vi "Dashboard Main.vi"() -> ()   [LabVIEW 2015]
uses:
  <vilib>/Utility/miscctls.llb/LVRowAndColumnTypeDef.ctl
  <vilib>/event_ctls.llb/eventvkey.ctl
  <vilib>/Rock Robotics/WPI/Dashboard/WPI_DashboardLogging Global.vi
  <vilib>/Rock Robotics/Network Tables/NT Read Numeric Array.vi
  <vilib>/Utility/config.llb/Write Key (String).vi
  <vilib>/Utility/config.llb/Write Key (I32).vi
  <vilib>/Utility/config.llb/NI_LVConfig.lvlib
panel:
  in  "TCP":refnum<k5>
  in  "Rec Mode":enum32{"Stop", "Record", "Playback"}(radio)
  in  "Vision":u16(ring)=1 items=["Camera Off", "USB Camera SW", "USB Camera HW", "IP Camera"]
  out "Camera IP":string
  out "Image Message":string="Timeout in Camera Communications"
  in  "Dashboard Tab":T1(tab)
  in  "Select Auto":string(combo)
  out "NT Connection":bool
  in  "Camera Settings":T2={"Frame Rate"=30, "Compression"=30, "Size"=1} {"Frame Rate" scale=1.0..30.0; "Size" items=["640x480", "320x240", "160x120"]}
  out "MotorChart R":cluster{"Numeric":dbl, "Numeric":dbl}(graph)
  out "MotorChart L":T3(graph)
  out "MotorSliders R":cluster{"MotorSlide1":dbl, "MotorSlide2":dbl} {"MotorSlide2" scale=-1.0..1.0 scale format="%#_2e"; "MotorSlide1" scale=-1.0..1.0 scale format="%#_2e"}
  out "MotorSliders L":T4 {"MotorSlide4 2" scale=0.0..14.0 scale format="%#_2e"; "MotorSlide2" scale=-1.0..1.0 scale format="%#_2e"; "MotorSlide1" scale=-1.0..1.0 scale format="%#_2e"}
  out "Gyro":dbl(knob) scale=0.0..360.0
  out "JS1 Z":dbl(slide) scale=-1.0..1.0 scale format="%#_2e"
  out "JS1 Graph":cluster{"X":dbl, "Y":dbl}[](graph)
  out "JS1 Buttons":T5
  out "JS2 Z":dbl(slide) scale=-1.0..1.0 scale format="%#_2e"
  out "JS2 Graph":cluster{"X":dbl, "Y":dbl}[](graph)
  out "JS2 Buttons":T5
  out "Mode":T6(ring)=enum."Auto Disabled"
  in  "DB Camera Config":bool
  out "fps":dbl format="%#.1g"
  out "Mbps":dbl format="%#.1g"
  out "Mbps LED":bool
  in  "DB/String 9":string
  in  "DB/String 8":string
  in  "DB/String 7":string
  in  "DB/String 6":string
  in  "DB/String 5":string
  in  "DB/String 4":string
  in  "DB/String 3":string
  in  "DB/String 2":string
  in  "DB/String 1":string
  in  "DB/String 0":string
  in  "DB/Slider 0":dbl(slide) scale=0.0..5.0
  in  "DB/Slider 1":dbl(slide) scale=0.0..5.0
  in  "DB/Slider 2":dbl(slide) scale=0.0..5.0
  in  "DB/Slider 3":dbl(slide) scale=0.0..5.0
  out "DB/LED 3":bool
  out "DB/LED 2":bool
  out "DB/LED 1":bool
  out "DB/LED 0":bool
  in  "DB/Button 3":bool
  in  "DB/Button 2":bool
  in  "DB/Button 1":bool
  in  "DB/Button 0":bool caption="New Name"
  in  "Top Wheel":dbl=-0.76
  in  "Bottom Wheel":dbl=0.6
  in  "tolerance":dbl=0.03
  in  "center":dbl=0.0125
  in  "higher speed":dbl=0.8
  in  "lower speed":dbl=0.67
  out "Vcenter":dbl
  out "Distances":dbl[](array[numeric])
  out "Hcenter":dbl
  in  "Left":i32=130
  in  "Top":i32=27
  in  "SquareSide":i32=40
  in  "Test Slider":dbl(slide) scale=0.0..100.0 scale format="%#_3g"
  in  "On/Off":bool caption="Solenoid"
  in  "Test Name":u16(ring) items=["Select the test to run..."]
  in  "Test Tree":string(tree)
  in  "Motor":cluster{"Value":dbl, "Enable":bool} {"Value" scale=-1.0..1.0 scale format="%#_3g"}
  out "Progress":T7 {"Test Progress" scale=0.0..100.0}
  in  "Rev/Fwd":cluster{"Forward":bool, "Reverse":bool}
  in  "Test Ring":u16(ring) items=["Monochrome", "Color"]
  out "Cmd Status":string
  in  "Execute Command":bool
  in  "Command Params":string[][](table)
  in  "Command Selection":i32(listbox)
  in  "CheckList":i32(listbox)
  out "Tree":string(tree)
  out "Camera Image":T8(plugin-control)
  out "Background":bool
  # "Left"
  # "Front"
  # "Right"
  # "Battery"
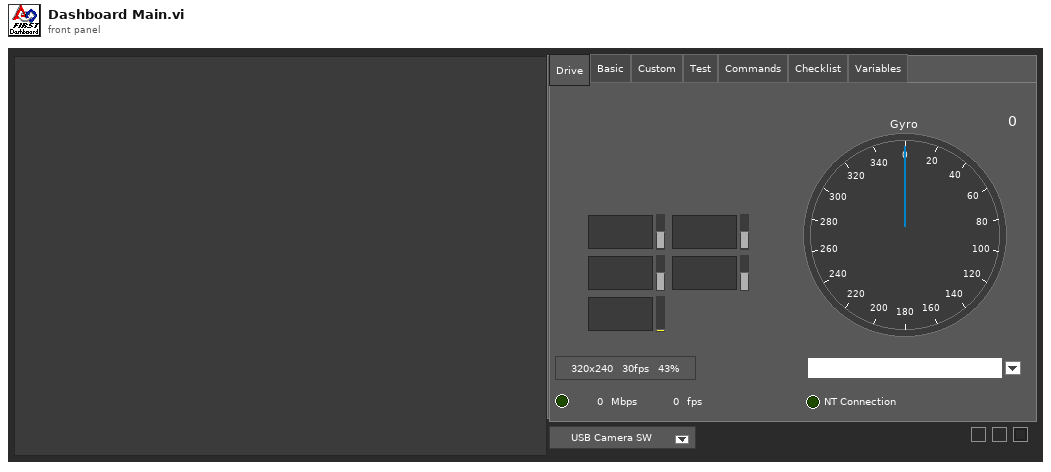
[diagram p1: front panel]
types:
  T1 = enum32{"Drive", "Basic", "Custom", "Test", "Commands", "Checklist", "Variables"}
  T2 = cluster{"Frame Rate":i32, "Compression":i32, "Size":u16}
  T3 = cluster{"Numeric":dbl, "Numeric":dbl, "Battery V":dbl}
  T4 = cluster{"MotorSlide1":dbl, "MotorSlide2":dbl, "MotorSlide4 2":dbl}
  T5 = cluster{bool, bool, bool, bool, bool, bool, bool, bool, bool, bool, bool, bool}
  T6 = enum8{"Tele-Op Disabled", "Tele-Op Enabled", "Auto Disabled", "Auto Enabled", "Test Disabled", "Test Enabled", "Disconnected", "No Code", "E-Stop"}
  T7 = cluster{"Test Progress":u8, "Test Progress Text":string}
  T8 = typedef "IMAQ Image.ctl" = refnum<image>
  T9 = cluster{"IDs":cluster{"RPC field ID":u16, "Unique ID":u16}, "String":string}
  T10 = enum32{"Drive", "Basic", "Custom", "Test", "Checklist", "Variables"}
  T11 = typedef "Image Type" = u32
  T12 = cluster{"Camera Image":refnum<vi>, "Dashboard Tab":refnum<vi>, "Background":refnum<vi>, "Vision":refnum<vi>, "Rec Mode":refnum<vi>, "Test Slider":refnum<vi>, "On/Off ":refnum<vi>, "Test Ring":refnum<vi>, "Rev/Fwd":refnum<vi>, "Test Name":refnum<vi>, "Motor":refnum<vi>, "Progress":refnum<vi>, "CheckList":refnum<vi>, "Tree":refnum<vi>, "Test Tree":refnum<vi>, "Command Params":refnum<vi>, "Command Selection":refnum<vi>, "Execute Command":refnum<vi>, "Cmd Status":refnum<vi>}
  T13 = cluster{"Error Strings":string, "Disable Counts":cluster{u16, u16}, "Rail Faults":cluster{u16, u16, u16}, "Robot IP":string, "DB Mode":u8, "Event Info":cluster{"Name":string, "Type":u8, "Number":u16, "Replay":u8}, "Camera Addr":string}
  T14 = cluster{"Storage":cluster{"Disk Free":u64, "RAM Block":u32, "RAM free":u32}, "CPU Utilization":cluster{"CPU % ISR":sgl, "CPU % Time Crit":sgl, "CPU % Timed Str":sgl, "CPU % High":sgl, "CPU % Above":sgl, "CPU % Normal":sgl, "CPU % Low":sgl}, "CAN":cluster{"% Bus Utilization":sgl, "Bus Off Cnt":u32, "TX_FIFO Full Cnt":u32, "Receive Error Cnt":u8, "Transmit Error Cnt":u8}, "HID":cluster{"HID Outputs":u32, "Rumble Low":u16, "Rumble High":u16}[]}
  T15 = cluster{"Status bits":cluster{"Test Mode":bool, "Autonomous":bool, "Enabled":bool, "Code Start":bool, "Brownout":bool, "Reserved 2":bool, "Reserved 3":bool, "E-Stop":bool}, "Code Trace":cluster{"Disabled":bool, "TeleOp":bool, "Auto":bool, "Test":bool}, "Controller Type":enum16{"unknown", "cRIO", "roboRio"}, "Code?":enum16{"unknown", "noCode", "code"}, "Battery V":dbl}
  T16 = cluster{"Control Bits":cluster{"TestMode":bool, "Autonomous":bool, "Enabled":bool, "FMS Present":bool, bool, bool, bool, "E-Stop":bool}, "Team Station ":u8, "Countdown":sgl, "Joystick Values":cluster{"Axes":dbl[], "Buttons":bool[], "POVs":i16[]}[]}
  T17 = cluster{"Axes":dbl[], "Buttons":bool[], "POVs":i16[]}[]
  T18 = cluster{"Axes":dbl[], "Buttons":bool[], "POVs":i16[]}
  T19 = cluster{"Buttons[0]":bool, "Buttons[1]":bool, "Buttons[2]":bool, "Buttons[3]":bool, "Buttons[4]":bool, "Buttons[5]":bool, "Buttons[6]":bool, "Buttons[7]":bool, "Buttons[8]":bool, "Buttons[9]":bool, "Buttons[10]":bool, "Buttons[11]":bool}
  T20 = typedef "NI_LVConfig.lvlib/Config Data RefNum.ctl" = refnum<k1>
  T21 = cluster{"Operation":enum16{"Update", "Clear"}, "Color Box":u32}[]
  T22 = typedef "eventvkey.ctl" = enum16{"ASCII", "Enter", "Return", "Shift", "Ctrl", "Alt", "Cmd", "Opt", "Caps", "NumLock", "Clear", "Break", "Up", "Down", "Left", "Right", "Insert", "Delete", "Home", "End", "PageUp", "PageDown", "Escape", "Help", "Pause", "ScrollLock", "F1", "F2", "F3", "F4", "F5", "F6", "F7", "F8", "F9", "F10", "F11", "F12", "F13", "F14", "F15", "F16", "F17", "F18", "F19", "F20", "F21", "F22", "F23", "F24", "Play", "VolumeUp", "VolumeDown", "Mute", "Two Byte Char"}
  T23 = cluster{"Image Size":bool, "Image Type":bool, "Pixel Value":bool, "ROI Information":bool, "Zoom Factor":bool}
  T24 = enum8{"Enabled", "Disabled", "Disabled and Grayed Out"}
  T25 = cluster{"Operation":enum16{"Update", "Clear"}, "Color Box":u32}
  T26 = typedef "LVRowAndColumnTypeDef.ctl" = cluster{"Row":i32, "Column":i32}
  T27 = cluster{"Shift":bool, "Ctrl":bool, "Alt":bool, "Cmd":bool, "Opt":bool}
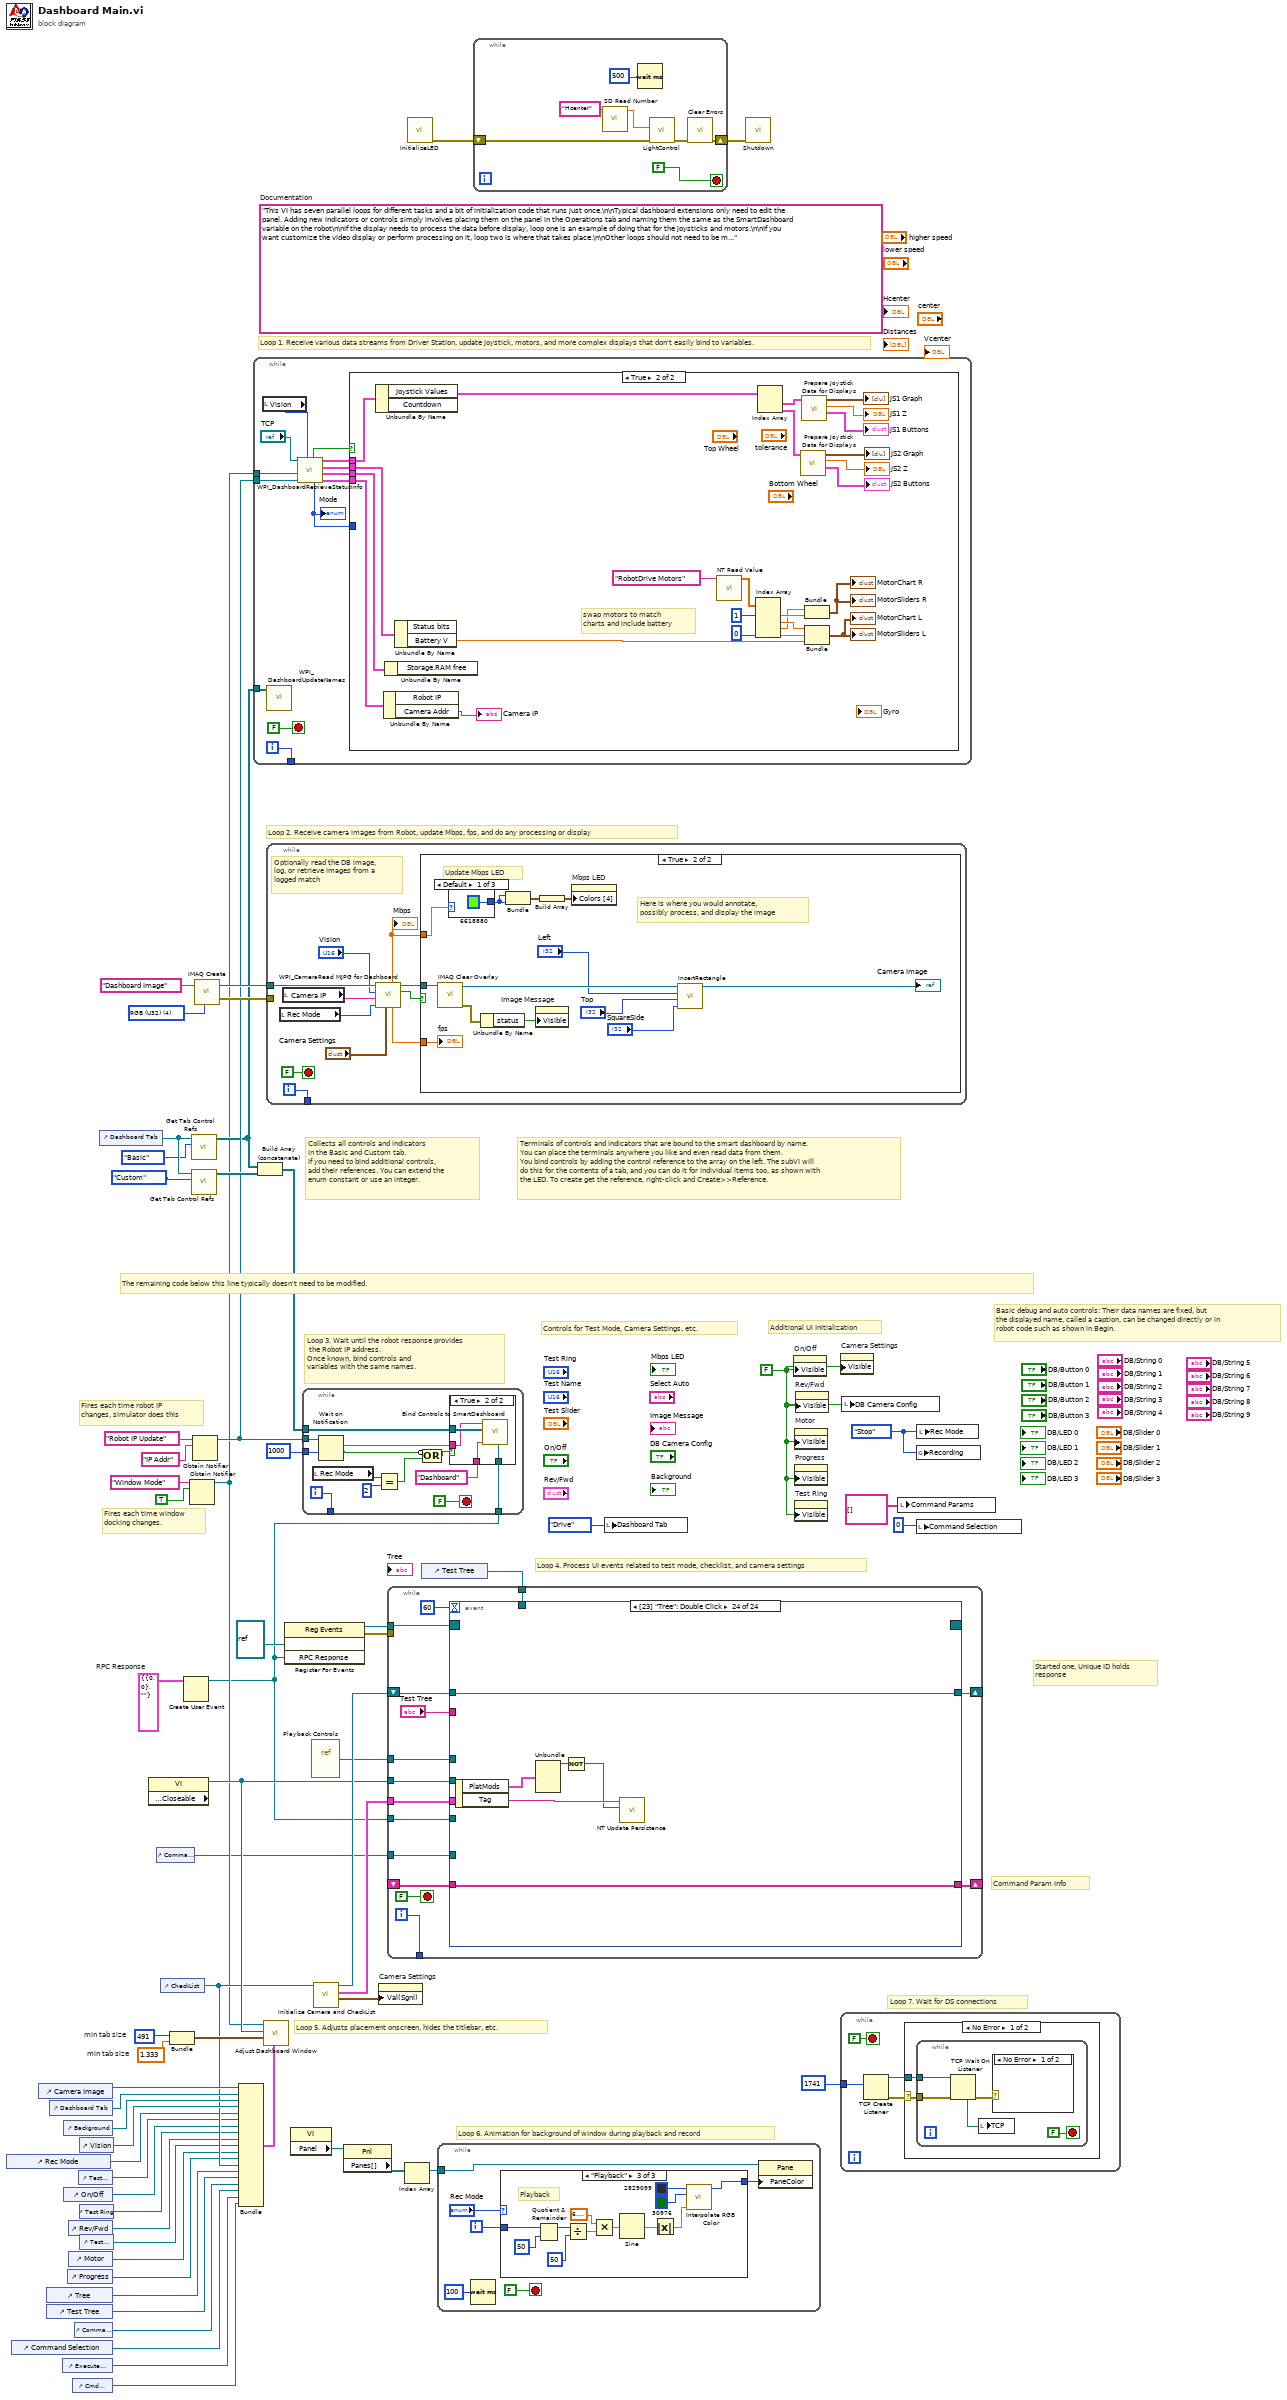
[diagram p0: block diagram]
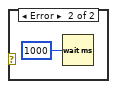
[diagram p2: hidden frame]
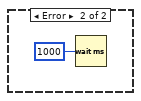
[diagram p3: hidden frame]
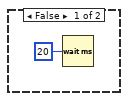
[diagram p4: hidden frame]
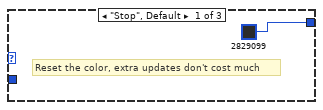
[diagram p5: hidden frame]
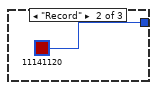
[diagram p6: hidden frame]
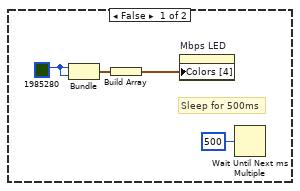
[diagram p8: hidden frame]
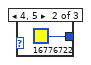
[diagram p9: hidden frame]
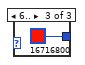
[diagram p10: hidden frame]
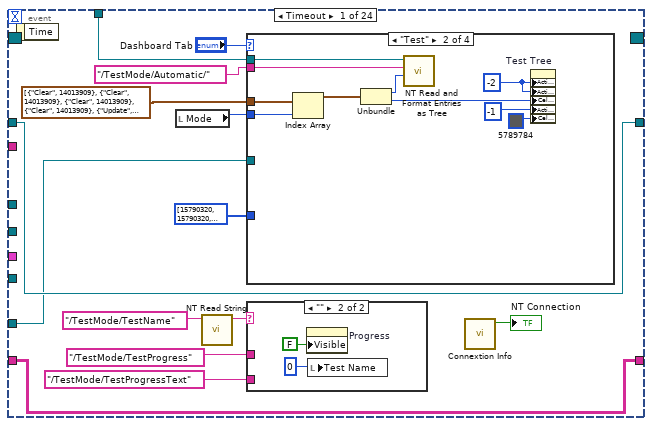
[diagram p11: hidden frame]
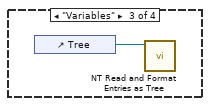
[diagram p13: hidden frame]
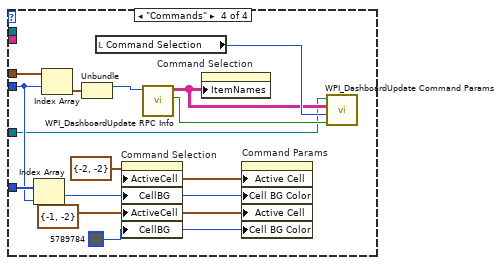
[diagram p14: hidden frame]
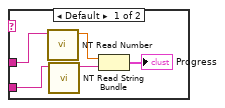
[diagram p15: hidden frame]
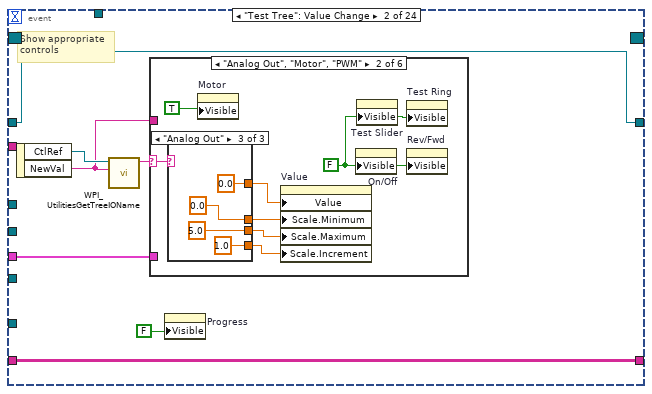
[diagram p16: hidden frame]
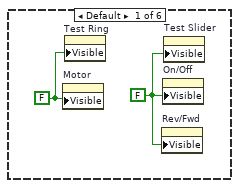
[diagram p17: hidden frame]
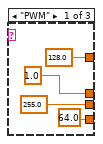
[diagram p18: hidden frame]
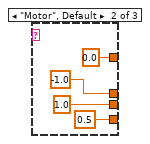
[diagram p19: hidden frame]
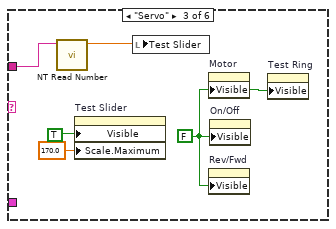
[diagram p20: hidden frame]
diagram:
  w9 = T9 {"IDs"={"RPC field ID"=0, "Unique ID"=0}, "String"=""}  # RPC Response
  w35 = 491  # min tab size
  w34 = 1.333  # min tab size
  w43 = enum32{"Stop", "Record", "Playback"}."Stop" ("Rec Mode")
  w17 = FALSE ("Visible")
  (unwired) "This VI has seven parallel loops for different tasks and a bit of initialization code that runs just once.\n\nTypical dashboard extensions only need to edit the panel. Adding new indicators or controls simply involves placing them on the panel in the Operations tab and naming them the same as the SmartDashboard variable on the robot\n\nIf the display needs to process the data before display, loop one is an example of doing that for the joysticks and motors.\n\nIf you want customize the video display or perform processing on it, loop two is where that takes place.\n\nOther loops should not need to be modified. They are pretty standard, and document the task they perform."  # Documentation
  w63 = T11 4 items=["Grayscale (U8)", "Grayscale (I16)", "Grayscale (SGL)", "Complex (CSG)", "RGB (U32)", "HSL (U32)", "RGB (U64)"] ("Image Type")
  # "Command Param Info"
  # "Started one, Unique ID holds\nresponse"
  # "Loop 7. Wait for DS connections"
  # "Basic debug and auto controls: Their data names are fixed, but\nthe displayed name, called a caption, can be changed directly or in\nrobot code such as shown in Begin."
  # "Controls for Test Mode, Camera Settings, etc."
  # "Additional UI Initialization"
  # "Loop 6. Animation for background of window during playback and record"
  # "Fires each time robot IP\nchanges, simulator does this"
  # "Fires each time window\ndocking changes."
  # "Collects all controls and indicators\nin the Basic and Custom tab.\nIf you need to bind additional controls,\nadd their references. You can extend the\nenum constant or use an integer."
  # "The remaining code below this line typically doesn't need to be modified."
  # "Loop 4. Process UI events related to test mode, checklist, and camera settings"
  # "Terminals of controls and indicators that are bound to the smart dashboard by name.\nYou can place the terminals anywhere you like and even read data from them.\nYou bind controls by adding the control reference to the array on the left. The subVI will\ndo this for the contents of a tab, and you can do it for individual items too, as shown with\nthe LED. To create get the reference, right-click and Create>>Reference."
  # "Loop 3. Wait until the robot response provides\n the Robot IP address.\nOnce known, bind controls and\nvariables with the same names."
  # "Loop 5. Adjusts placement onscreen, hides the titlebar, etc."
  # "Loop 1. Receive various data streams from Driver Station, update joystick, motors, and more complex displays that don't easily bind to variables."
  # "Loop 2. Receive camera images from Robot, update Mbps, fps, and do any processing or display"
  n1 = control-ref of="Rec Mode"() -> (w23:refnum<vi>)
  n2 = control-ref of="Command Selection"() -> (w8:refnum<vi>)
  n3 = control-ref of="Camera Image"() -> (w38:refnum<vi>)
  n4 = control-ref of="Tree"() -> (w27:refnum<vi>)
  n5 = control-ref of="Test Tree"() -> (w26:refnum<vi>)
  n6 = control-ref of="Dashboard Tab"() -> (w37:refnum<vi>)
  n7 = control-ref of="Execute Command"() -> (w10:refnum<vi>)
  n8 = control-ref of="Background"() -> (w32:refnum<vi>)
  n9 = control-ref of="On/Off"() -> (w21:refnum<vi>)
  n10 = control-ref of="Progress"() -> (w18:refnum<vi>)
  n11 = control-ref of="Rev/Fwd"() -> (w19:refnum<vi>)
  n12 = control-ref of="Motor"() -> (w24:refnum<vi>)
  n13 = control-ref of="Cmd Status"() -> (w4:refnum<vi>)
  n14 = control-ref of="Command Params"() -> (w11:refnum<vi>)
  n15 = control-ref of="Test Slider"() -> (w22:refnum<vi>)
  n16 = control-ref of="Vision"() -> (w36:refnum<vi>)
  n17 = control-ref of="Test Ring"() -> (w20:refnum<vi>)
  n18 = control-ref of="Test Name"() -> (w25:refnum<vi>)
  n19 = control-ref of="Dashboard Tab"() -> (w41:refnum<vi>)
  n20 = property class="VI" props=["Front Panel.Closeable"]() -> (reference out=w42:refnum<vi>)  [unwired: 2 in, 2 out]
  n21 = control-ref of="Command Params"() -> (w3:refnum<vi>)
  n22 = control-ref of="CheckList"() -> (w28:refnum<vi>)
  n23 = Bundle("min tab size"=w35, "min tab size"=w34) -> (w33:cluster{"min tab size":i32, "min tab size":dbl})  [unwired: 1 in]
  n24 = Create User Event(user event datatype=w9) -> (user event=w5:refnum<user-event>)  [unwired: 1 in, 1 out]
  n25 = Obtain Notifier(name (unnamed)="Window Mode", notification data type=TRUE) -> (notifier out=w14:refnum<notifier>)  [unwired: 2 in, 2 out]
  n26 = call <vilib>:"Get Tab Control Refs.vi"("Page Index"=T10."Basic" ("Dashboard Tab"), "TabControl in"=w41) -> ("ControlsOnPage"=w15:refnum<vi>[])  [unwired: 9 in]
  n27 = call <vilib>:"Get Tab Control Refs.vi"("Page Index"=T10."Custom" ("Dashboard Tab"), "TabControl in"=w41) -> ("ControlsOnPage"=w40:refnum<vi>[])  [unwired: 9 in]
  n28 = Obtain Notifier(name (unnamed)="Robot IP Update", notification data type="IP Addr" ("name (unnamed)")) -> (notifier out=w16:refnum<notifier>)  [unwired: 2 in, 2 out]
  n29 = call "IMAQ Create"("Image Name"="Dashboard Image", "Image Type"=w63) -> ("New Image"=w61:T8, "error out"=w60:errorcluster)  [unwired: 2 in, 1 out]
  n30 = Bundle("Camera Image"=w38, "Dashboard Tab"=w37, "Background"=w32, "Vision"=w36, "Rec Mode"=w23, "Test Slider"=w22, "On/Off"=w21, "Test Ring"=w20, "Rev/Fwd"=w19, "Test Name"=w25, "Motor"=w24, "Progress"=w18, "CheckList"=w28, "Tree"=w27, "Test Tree"=w26, "Command Params"=w11, "Command Selection"=w8, "Execute Command"=w10, "Cmd Status"=w4) -> (w29:T12)  [unwired: 1 in]
  n31 = while {
    tunnel: [w75] -> _
    tunnel: w16 -> [w69]
    tunnel: w15 -> [w68]
    tunnel: w14 -> [w64]
    i -> [w75]
    stop <- FALSE stop-if-true
    n32 = local read "Vision"() -> (w66:u16)
    n33 = call <vilib>:"WPI_DashboardUpdateNames.vi"("Controls on Tab"=w68) -> ()  [unwired: 11 in]
    n34 = call <vilib>:"WPI_DashboardRetrieveStatusInfo.vi"("Vision"=w66, "Binding Refnum"=w69, "Window Mode Notifier"=w64, "TCP Cnx"="TCP") -> ("Power and Errors"=w70:T13, "Robot Metrics"=w73:T14, "Status Info"=w74:T15, "Control Info"=w71:T16, "Robot Mode"=w67:T6, "Process?"=w72:bool)  [unwired: 2 in]
    "Mode" <- w67
    n35 = case shown="True" w72 {
      tunnel: w74 -> [_ w102]
      tunnel: w73 -> [_ w101]
      tunnel: w71 -> [_ w100]
      tunnel: w70 -> [_ w99]
      tunnel: w67 -> [_ _]
      frame False {
        n36 = Wait (ms)(milliseconds to wait=u32 20) -> ()  [unwired: 1 out]
      }
      frame True {
        # "swap motors to match\ncharts and include battery"
        n37 = Unbundle By Name(w100) -> ("Joystick Values"=w89:T17)  [unwired: 1 out]
        n38 = Unbundle By Name(w99) -> ("Camera Addr"=→"Camera IP":string)  [unwired: 1 out]
        n39 = Unbundle By Name(w101) -> ()  [unwired: 1 out]
        n40 = Unbundle By Name(w102) -> ("Battery V"=w90:dbl)  [unwired: 1 out]
        n41 = call-poly <vilib>:"NT Read Value.vi"("Name"="RobotDrive Motors") -> ("Numeric Array"=w78:dbl[])  [unwired: 9 in, 1 out]
        n42 = Index Array(array=w78, index #1=1, index #4=0) -> (element #1=w94:dbl, element #2=w95:dbl, element #3=w93:dbl, element #4=w98:dbl)  [unwired: 2 in]
        n43 = Index Array(array=w89) -> (element #1=w88:T18, element #2=w83:T18)  [unwired: 2 in]
        n44 = call "Prepare Joystick Data for Displays.vi"("Joystick Values"=w83) -> ("Buttons"=→"JS2 Buttons":T19, "Z Axis"=→"JS2 Z":dbl, "Cartesian Data"=→"JS2 Graph":cluster{"X axis":dbl, "X axis":dbl}[])  [unwired: 8 in]
        n45 = call "Prepare Joystick Data for Displays.vi"("Joystick Values"=w88) -> ("Buttons"=→"JS1 Buttons":T19, "Z Axis"=→"JS1 Z":dbl, "Cartesian Data"=→"JS1 Graph":cluster{"X axis":dbl, "X axis":dbl}[])  [unwired: 8 in]
        n46 = Bundle("Numeric"=w93, "Numeric"=w94) -> (→"MotorChart R" →"MotorSliders R":cluster{"Numeric":dbl, "Numeric":dbl})  [unwired: 1 in]
        n47 = Bundle("Numeric"=w95, "Numeric"=w98, "Battery V"=w90) -> (→"MotorChart L" →"MotorSliders L":T3)  [unwired: 1 in]
      }
    }
  }
  n48 = Build Array (concatenate)(w15, w40) -> (w39:refnum<vi>[])
  n49 = call "Adjust Dashboard Window.vi"("Sizing Refnums"=w29, "Size Constraints"=w33, "VI"=w42, "WIn Mode"=w14) -> ()  [unwired: 8 in]
  n50 = while {
    tunnel: w61 -> [w111]
    tunnel: w60 -> [_]
    tunnel: [w112] -> _
    i -> [w112]
    stop <- FALSE stop-if-true
    # "Optionally read the DB image,\nlog, or retrieve images from a\nlogged match"
    n51 = local read "Rec Mode"() -> (w106:enum32{"Stop", "Record", "Playback"})
    n52 = local read "Camera IP"() -> (w104:string)
    n53 = call <vilib>:"WPI_CameraRead MJPG for Dashboard.vi"("Camera Settings"="Camera Settings", "Rec Mode"=w106, "Camera IP"=w104, "Camera Mode"="Vision", "Refnum in"=w111) -> ("Active"=w109:bool, "Refnum out"=w110:T8, "FPS"=w108:dbl, "Bandwidth (Mbps)"=w103:dbl)  [unwired: 3 in]
    "Mbps" <- w103
    n54 = case shown="True" w109 {
      tunnel: w110 -> [_ w125]
      tunnel: w103 -> [_ w124]
      tunnel: w108 -> [_ w123]
      frame False {
        w114 = u32 1985280 ("Color Box")
        # "Sleep for 500ms"
        n55 = Bundle("Color Box"=w114, "Color Box"=w114) -> (w116:cluster{"Color Box":u32, "Color Box":u32})  [unwired: 1 out]
        n56 = Build Array(w116) -> (w115:cluster{"Color Box":u32, "Color Box":u32}[])
        n57 = property on="Mbps LED" class="Bool (strict)"("Colors [4]"=w115) -> ()  [unwired: 2 in, 2 out]
        n58 = Wait Until Next ms Multiple(millisecond multiple=u32 500) -> ()  [unwired: 1 out]
      }
      frame True {
        # "Here is where you would annotate,\npossibly process, and display the image"
        # "Update Mbps LED"
        n59 = call "IMAQ Clear Overlay"("Image"=w125) -> ("error out"=w129:errorcluster, "Image Out"=w122:T8)  [unwired: 2 in, 7 out]
        n60 = case shown="Default" w124 {
          tunnel: [u32 6618880 ("Color Box") u32 16776722 ("Color Box") u32 16716800 ("Color Box")] -> w126
          frame Default {
          }
          frame 4, 5 {
          }
          frame 6.. {
          }
        }
        n61 = Unbundle By Name(w129) -> ("status"=w130:bool)
        n62 = Bundle("Color Box"=w126, "Color Box"=w126) -> (w128:cluster{"Color Box":u32, "Color Box":u32})  [unwired: 1 out]
        n63 = property on="Image Message" class="Str"("Visible"=w130) -> ()  [unwired: 2 in, 2 out]
        n64 = Build Array(w128) -> (w127:cluster{"Color Box":u32, "Color Box":u32}[])
        n65 = property on="Mbps LED" class="Bool (strict)"("Colors [4]"=w127) -> ()  [unwired: 2 in, 2 out]
        n66 = call "InsertRectangle.vi"("SquareSide"="SquareSide", "Top"="Top", "Left"="Left", "Refnum in"=w122) -> ("Refnum out"=→"Camera Image":T8)  [unwired: 7 in]
        "fps" <- w123
      }
    }
  }
  n67 = register-events(refnum<vi> refnum, w5) -> (reference out=w47:refnum<event-registration>, error out=w46:errorcluster)  [unwired: 2 in]
  n68 = property class="VI"() -> ("Panel"=w50:refnum<vi>)  [unwired: 2 in, 2 out]
  n69 = while {
    tunnel: w39 -> [w146]
    tunnel: w16 -> [w144]
    tunnel: [w142] -> _
    tunnel: u32 1000 ("milliseconds to wait") -> [w141]
    tunnel: w5 -> [w134]
    i -> [w142]
    stop <- FALSE stop-if-true
    n70 = local read "Rec Mode"() -> (w137:enum32{"Stop", "Record", "Playback"})
    n71 = Wait on Notification(notifier=w144, timeout in ms (-1)=w141) -> (notification=w143:string, timed out?=w139:bool)  [unwired: 2 in, 2 out]
    n72 = Equal?(x=w137, y=u16 2 ("Rec Mode")) -> (x = y?=w138:bool)
    n73 = Compound Arithmetic op=OR(invert w139, w138) -> (w140:bool)
    n74 = case shown="True" w140 {
      tunnel: w146 -> [_ w150]
      tunnel: w143 -> [_ w149]
      tunnel: "Dashboard" -> [_ w148]
      tunnel: w134 -> [_ w147]
      frame False {
      }
      frame True {
        n75 = call <vilib>:"Bind Controls to SmartDashboard.vi"("RPC ref"=w147, "Client Name"=w148, "Bound Control Refs"=w150, "Server IP Address"=w149) -> ()  [unwired: 8 in]
      }
    }
  }
  n76 = vi-ref "Playback Controls.vi"() -> (w48:refnum<vi>)
  n77 = call "Initialize Camera and CheckList.vi"("ListBox in"=w28) -> ("Cluster"=w54:cluster{"value":i32, "value":i32, "index":i32}, "Array"=w55:cluster{string[]}[], "File Refnum"=w53:T20)  [unwired: 8 in]
  n78 = property class="Pnl"(reference=w50) -> ("Panes[]"=w51:refnum<vi>[])  [unwired: 1 in, 2 out]
  n79 = property on="Camera Settings" class="Clust (strict)"("Val(Sgnl)"=w54) -> ()  [unwired: 2 in, 2 out]
  n80 = Index Array(array=w51) -> (element=w49:refnum<vi>)  [unwired: 1 in]
  n81 = call "InitializeLED.vi"() -> ("error out"=w1:errorcluster)  [unwired: 11 in]
  n82 = control-ref of="Test Tree"() -> (w52:refnum<vi>)
  n83 = while {
    tunnel: w55 -> [w162]
    shift-right: [w161] -> _
    shift-left: w53 -> [w160]
    tunnel: [w159] -> _
    tunnel: w52 -> [w158]
    tunnel: w48 -> [w157]
    tunnel: w47 -> [w156]
    tunnel: w46 -> [_]
    tunnel: w42 -> [w155]
    tunnel: w5 -> [w154]
    tunnel: w3 -> [w153]
    shift-right: [w152] -> _
    shift-left: _ -> [w151]
    i -> [w159]
    stop <- FALSE stop-if-true
    n84 = event shown="[23] \"Tree\": Double Click" {
      selector: w156 -> [_ _ _ _ _ _ _ _ _ _ _ _ _ _ _ _ _ _ _ _ _ _ _ _]
      dyn-events: [_ _ _ _ _ _ _ _ _ _ _ _ _ _ _ _ _ _ w471 _ _ _ _ _] -> _
      timeout: u32 60 ("milliseconds to wait") -> [_ _ _ _ _ _ _ _ _ _ _ _ _ _ _ _ _ _ _ _ _ _ _ _]
      tunnel: w158 -> [w175 _ _ _ _ _ _ _ _ _ _ _ _ _ _ _ _ _ _ _ _ _ _ _]
      tunnel: "Test Tree" -> [_ _ _ _ _ _ _ _ _ _ _ _ _ w434 w443 w446 w451 w460 _ _ _ _ _ _]
      tunnel: w162 -> [_ w213 _ _ _ _ _ _ _ _ _ w396 w427 _ _ _ _ _ _ _ _ _ _ _]
      tunnel: [w172 w212 w316 w322 w332 w336 w342 w354 w362 w368 w381 w395 w420 w433 w441 w445 w450 w459 w473 w489 w491 w499 w510 w515] -> w161
      tunnel: w160 -> [w172 w212 w316 w322 w332 w336 w342 w354 w362 w368 w381 w394 w420 w433 w441 w445 w450 w459 w473 w489 w491 w499 w510 w515]
      tunnel: w157 -> [_ _ _ _ _ _ _ _ _ _ _ _ _ _ _ _ _ _ w474 _ w494 _ _ _]
      tunnel: w155 -> [_ _ _ _ _ _ _ _ _ _ _ _ _ _ _ _ _ _ w469 _ _ _ _ _]
      tunnel: w154 -> [_ _ _ _ _ _ _ _ _ _ _ _ _ _ _ _ _ _ w465 _ _ _ _ _]
      tunnel: w153 -> [w167 _ _ _ _ _ w340 _ _ _ _ _ _ _ _ _ _ _ _ _ _ _ _ _]
      tunnel: [w166 w211 w315 w321 w331 w337 w338 w348 w359 w367 w380 w393 w419 w432 w440 w444 w449 w458 w464 w487 w490 w495 w503 w516] -> w152
      tunnel: w151 -> [w166 w211 w315 w321 w331 w337 w338 _ _ w367 w380 w393 w419 w432 w440 w444 w449 w458 w464 w487 w490 w495 w503 w516]
      event Timeout {
        n85 = event-data() -> ()  [unwired: 1 in, 1 out]
        n86 = local read "Mode"() -> (w169:T6)
        n87 = call <vilib>:"NT Read String.vi"("Name"="/TestMode/TestName") -> ("String"=w178:string)  [unwired: 9 in, 1 out]
        n88 = case shown="\"Test\"" "Dashboard Tab" {
          tunnel: w175 -> [_ w189 _ _]
          tunnel: "/TestMode/Automatic/" ("Name Pattern") -> [_ w188 _ _]
          tunnel: T21 [{"Operation"=enum."Clear", "Color Box"=14013909}, {"Operation"=enum."Clear", "Color Box"=14013909}, {"Operation"=enum."Clear", "Color Box"=14013909}, {"Operation"=enum."Clear", "Color Box"=14013909}, {"Operation"=enum."Update", "Color Box"=14013909}, {"Operation"=enum."Update", "Color Box"=16777215}, {"Operation"=enum."Clear", "Color Box"=14013909}, {"Operation"=enum."Clear", "Color Box"=14013909}, {"Operation"=enum."Clear", "Color Box"=14013909}] -> [_ w181 _ w198]
          tunnel: w169 -> [_ w180 _ w197]
          tunnel: u32[] [15790320, 15790320, 15790320, 15790320, 16777215, 16777215, 15790320, 15790320, 15790320] -> [_ _ _ w203]
          tunnel: w167 -> [_ _ _ w191]
          frame "Custom", Default {
          }
          frame "Test" {
            w187 = -2 ("Active Item:Row Number")
            n89 = Index Array(array=w181, index=w180) -> (element=w182:T25)
            n90 = Unbundle(w182) -> ("Operation"=w183:enum16{"Update", "Clear"}, "Color Box"=w184:u32)
            n91 = call <vilib>:"NT Read and Format Entries as Tree.vi"("Operation"=w183, "Name Pattern"=w188, "Tree Refnum"=w189) -> ()  [unwired: 7 in, 2 out]
            n92 = property on="Test Tree" class="Tree (strict)"("Active Item Row Number"=w187, "ActiveColNum"=w187, "CellBG"=w184, "Active Item Row Number"=-1 ("Active Item:Row Number"), "CellBG"=u32 5789784 ("Color Box")) -> ()  [unwired: 2 in, 2 out]
          }
          frame "Variables" {
            n93 = control-ref of="Tree"() -> (w190:refnum<vi>)
            n94 = call <vilib>:"NT Read and Format Entries as Tree.vi"("Tree Refnum"=w190) -> ()  [unwired: 9 in, 2 out]
          }
          frame "Commands" {
            w199 = u32 5789784 ("Color Box")
            w200 = T26 {"Row"=-1, "Column"=-2} ("Active Cell:Active Cell")
            w202 = T26 {"Row"=-2, "Column"=-2} ("Active Cell:Active Cell")
            n95 = Index Array(array=w203, index=w197) -> (element=w201:u32)
            n96 = Index Array(array=w198, index=w197) -> (element=w196:T25)
            n97 = Unbundle(w196) -> ("Operation"=w195:enum16{"Update", "Clear"})  [unwired: 1 out]
            n98 = local read "Command Selection"() -> (w194:i32)
            n99 = property on="Command Selection" class="MCListbox (strict)"("ActiveCell"=w202, "CellBG"=w201, "ActiveCell"=w200, "CellBG"=w199) -> ()  [unwired: 2 in, 2 out]
            n100 = call <vilib>:"WPI_DashboardUpdate RPC Info.vi"("Operation"=w195) -> ("update"=w193:bool, "commands"=w192:string[][])  [unwired: 9 in]
            n101 = property on="Command Selection" class="MCListbox (strict)"("ItemNames"=w192) -> ()  [unwired: 2 in, 2 out]
            n102 = property on="Command Params" class="Tbl (strict)"("Active Cell"=w202, "Cell BG Color"=w201, "Active Cell"=w200, "Cell BG Color"=w199) -> ()  [unwired: 2 in, 2 out]
            n103 = call <vilib>:"WPI_DashboardUpdate Command Params.vi"("Update"=w193, "NewVal"=w194, "Commands"=w192, "Param Tbl"=w191) -> ()  [unwired: 7 in, 1 out]
          }
        }
        n104 = case shown="\"\"" w178 {
          tunnel: "/TestMode/TestProgress" ("Name") -> [w205 _]
          tunnel: "/TestMode/TestProgressText" ("Name") -> [w204 _]
          frame Default {
            n105 = call <vilib>:"NT Read Number.vi"("Name"=w205) -> ("Numeric"=w206:dbl)  [unwired: 9 in, 1 out]
            n106 = call <vilib>:"NT Read String.vi"("Name"=w204) -> ("String"=w207:string)  [unwired: 9 in, 1 out]
            n107 = Bundle("Numeric"=w206, "String"=w207) -> (→"Progress":cluster{"Numeric":dbl, "String":string})  [unwired: 1 in]
          }
          frame "" {
            n108 = property on="Progress" class="Clust (strict)"("Visible"=FALSE) -> ()  [unwired: 2 in, 2 out]
            n109 = local write "Test Name"(u16 0) -> ()
          }
        }
        n110 = call <vilib>:"Connextion Info.vi"() -> ("Connected"=→"NT Connection":bool)  [unwired: 10 in, 1 out]
      }
      event "Test Tree": Value Change {
        # "Show appropriate\ncontrols"
        n111 = event-data() -> ("CtlRef"=w216:refnum<vi>, "NewVal"=w214:string)  [unwired: 1 in]
        n112 = call <vilib>:"WPI_UtilitiesGetTreeIOName.vi"("NewVal"=w214, "TreeControl in"=w216) -> ("I/O Name"=w217:string)  [unwired: 9 in]
        n113 = case shown="\"Analog Out\", \"Motor\", \"PWM\"" w217 {
          selector: w217 -> [_ w224 _ w246 w255 _]
          tunnel: w214 -> [_ _ w243 w245 _ w262]
          tunnel: w213 -> [_ _ _ _ _ w261]
          frame Default {
            w219 = FALSE ("Visible")
            w218 = FALSE ("Visible")
            n114 = property on="Motor" class="Clust (strict)"("Visible"=w218) -> ()  [unwired: 2 in, 2 out]
            n115 = property on="Test Ring" class="Ring (strict)"("Visible"=w218) -> ()  [unwired: 2 in, 2 out]
            n116 = property on="Rev/Fwd" class="Clust (strict)"("Visible"=w219) -> ()  [unwired: 2 in, 2 out]
            n117 = property on="On/Off" class="Bool (strict)"("Visible"=w219) -> ()  [unwired: 2 in, 2 out]
            n118 = property on="Test Slider" class="Slide (strict)"("Visible"=w219) -> ()  [unwired: 2 in, 2 out]
          }
          frame "Analog Out", "Motor", "PWM" {
            w225 = FALSE ("Visible")
            n119 = case shown="\"Analog Out\"" w224 {
              tunnel: [1.0 ("Value") -1.0 ("Value") 0.0 ("Value")] -> w223
              tunnel: [255.0 ("Value") 1.0 ("Value") 5.0 ("Value")] -> w222
              tunnel: [128.0 ("Value") 0.0 ("Value") 0.0 ("Value")] -> w221
              tunnel: [64.0 ("Value") 0.5 ("Value") 1.0 ("Value")] -> w220
              frame "PWM" {
              }
              frame "Motor", Default {
              }
              frame "Analog Out" {
              }
            }
            n120 = property on="Motor" class="Clust (strict)"("Visible"=TRUE) -> ()  [unwired: 2 in, 2 out]
            n121 = property on="Value" class="Slide (strict)"("Value"=w221, "Scale.Minimum"=w223, "Scale.Maximum"=w222, "Scale.Increment"=w220) -> ()  [unwired: 2 in, 2 out]
            n122 = property on="On/Off" class="Bool (strict)"("Visible"=w225) -> ()  [unwired: 2 in, 2 out]
            n123 = property on="Test Slider" class="Slide (strict)"("Visible"=w225) -> ()  [unwired: 2 in, 2 out]
            n124 = property on="Test Ring" class="Ring (strict)"("Visible"=w225) -> ()  [unwired: 2 in, 2 out]
            n125 = property on="Rev/Fwd" class="Clust (strict)"("Visible"=w225) -> ()  [unwired: 2 in, 2 out]
          }
          frame "Servo" {
            w241 = FALSE ("Visible")
            n126 = call <vilib>:"NT Read Number.vi"("Name"=w243) -> ("Numeric"=w242:dbl)  [unwired: 9 in, 1 out]
            n127 = property on="Test Slider" class="Slide (strict)"("Visible"=TRUE, "Scale.Maximum"=170.0 ("Scale.Range:Maximum")) -> ()  [unwired: 2 in, 2 out]
            n128 = local write "Test Slider"(w242) -> ()
            n129 = property on="Motor" class="Clust (strict)"("Visible"=w241) -> ()  [unwired: 2 in, 2 out]
            n130 = property on="Rev/Fwd" class="Clust (strict)"("Visible"=w241) -> ()  [unwired: 2 in, 2 out]
            n131 = property on="On/Off" class="Bool (strict)"("Visible"=w241) -> ()  [unwired: 2 in, 2 out]
            n132 = property on="Test Ring" class="Ring (strict)"("Visible"=w241) -> ()  [unwired: 2 in, 2 out]
          }
          frame "Relay", "Solenoid" {
            w244 = FALSE ("Visible")
            n133 = property on="Motor" class="Clust (strict)"("Visible"=w244) -> ()  [unwired: 2 in, 2 out]
            n134 = property on="Test Slider" class="Slide (strict)"("Visible"=w244) -> ()  [unwired: 2 in, 2 out]
            n135 = Search and Replace String(input string=w245, search string="/Value  **", replace string="/Direction") -> (result string=w251:string)  [unwired: 5 in, 3 out]
            n136 = property on="Test Ring" class="Ring (strict)"("Visible"=w244) -> ()  [unwired: 2 in, 2 out]
            n137 = call <vilib>:"NT Read String.vi"("Name"=w251) -> ("String"=w249:string)  [unwired: 9 in, 1 out]
            n138 = Equal?(x="Both directions", y=w249) -> (x = y?=w247:bool)
            n139 = Not(x=w247) -> (.not. x?=w248:bool)
            n140 = property on="Rev/Fwd" class="Clust (strict)"("Visible"=w247) -> ()  [unwired: 2 in, 2 out]
            n141 = property on="On/Off" class="Bool (strict)"("Visible"=w248, "Caption.Text"=w246) -> ()  [unwired: 2 in, 2 out]
          }
          frame "Compressor", "Digital Out" {
            w254 = FALSE ("Visible")
            # "Get direction and finish"
            n142 = property on="Motor" class="Clust (strict)"("Visible"=w254) -> ()  [unwired: 2 in, 2 out]
            n143 = property on="Test Slider" class="Slide (strict)"("Visible"=w254) -> ()  [unwired: 2 in, 2 out]
            n144 = property on="Test Ring" class="Ring (strict)"("Visible"=w254) -> ()  [unwired: 2 in, 2 out]
            n145 = property on="On/Off" class="Bool (strict)"("Visible"=TRUE, "Caption.Text"=w255) -> ()  [unwired: 2 in, 2 out]
            n146 = property on="Rev/Fwd" class="Clust (strict)"("Visible"=FALSE) -> ()  [unwired: 2 in, 2 out]
          }
          frame "Camera" {
            n147 = call <vilib>:"Get Last Path Segment.vi"("String in"=w262) -> ("String out"=w263:string)  [unwired: 10 in]
            n148 = property on="On/Off" class="Bool (strict)"("Visible"=FALSE) -> ()  [unwired: 2 in, 2 out]
            n149 = property on="Motor" class="Clust (strict)"("Visible"=FALSE) -> ()  [unwired: 2 in, 2 out]
            n150 = property on="Rev/Fwd" class="Clust (strict)"("Visible"=FALSE) -> ()  [unwired: 2 in, 2 out]
            n151 = case shown="\"White Balance  **\"" w263 {
              tunnel: w262 -> [w269 w278 w287 w296 w305 _ w311]
              tunnel: w261 -> [w267 w275 w284 w293 w302 _ _]
              frame "Size  **" {
                n152 = Index Array(array=w267) -> (element=w266:cluster{string[]})  [unwired: 1 in]
                n153 = call <vilib>:"NT Read String.vi"("Name"=w269) -> ("String"=w268:string)  [unwired: 9 in, 1 out]
                n154 = Unbundle(w266) -> (w264:string[])
                n155 = Match First String(2:w264, 3:w268) -> (0:w265:i32)  [unwired: 1 out]
                n156 = property on="Test Ring" class="Ring (strict)"("Value"=w265, "Strings []"=w264) -> ()  [unwired: 2 in, 2 out]
                n157 = property on="Test Ring" class="Ring (strict)"("Visible"=TRUE) -> ()  [unwired: 2 in, 2 out]
                n158 = property on="Test Slider" class="Slide (strict)"("Visible"=FALSE) -> ()  [unwired: 2 in, 2 out]
              }
              frame "White Balance  **" {
                n159 = Index Array(array=w275, index=1) -> (element=w276:cluster{string[]})
                n160 = call <vilib>:"NT Read String.vi"("Name"=w278) -> ("String"=w277:string)  [unwired: 9 in, 1 out]
                n161 = Unbundle(w276) -> (w273:string[])
                n162 = Match First String(2:w273, 3:w277) -> (0:w272:i32)  [unwired: 1 out]
                n163 = property on="Test Ring" class="Ring (strict)"("Value"=w272, "Strings []"=w273) -> ()  [unwired: 2 in, 2 out]
                n164 = property on="Test Ring" class="Ring (strict)"("Visible"=TRUE) -> ()  [unwired: 2 in, 2 out]
                n165 = property on="Test Slider" class="Slide (strict)"("Visible"=FALSE) -> ()  [unwired: 2 in, 2 out]
              }
              frame "Exposure  **" {
                n166 = Index Array(array=w284, index=2) -> (element=w285:cluster{string[]})
                n167 = call <vilib>:"NT Read String.vi"("Name"=w287) -> ("String"=w286:string)  [unwired: 9 in, 1 out]
                n168 = Unbundle(w285) -> (w281:string[])
                n169 = Match First String(2:w281, 3:w286) -> (0:w282:i32)  [unwired: 1 out]
                n170 = property on="Test Ring" class="Ring (strict)"("Value"=w282, "Strings []"=w281) -> ()  [unwired: 2 in, 2 out]
                n171 = property on="Test Ring" class="Ring (strict)"("Visible"=TRUE) -> ()  [unwired: 2 in, 2 out]
                n172 = property on="Test Slider" class="Slide (strict)"("Visible"=FALSE) -> ()  [unwired: 2 in, 2 out]
              }
              frame "Exposure Priority  **" {
                n173 = Index Array(array=w293, index=3) -> (element=w294:cluster{string[]})
                n174 = call <vilib>:"NT Read String.vi"("Name"=w296) -> ("String"=w295:string)  [unwired: 9 in, 1 out]
                n175 = Unbundle(w294) -> (w290:string[])
                n176 = Match First String(2:w290, 3:w295) -> (0:w291:i32)  [unwired: 1 out]
                n177 = property on="Test Ring" class="Ring (strict)"("Value"=w291, "Strings []"=w290) -> ()  [unwired: 2 in, 2 out]
                n178 = property on="Test Ring" class="Ring (strict)"("Visible"=TRUE) -> ()  [unwired: 2 in, 2 out]
                n179 = property on="Test Slider" class="Slide (strict)"("Visible"=FALSE) -> ()  [unwired: 2 in, 2 out]
              }
              frame "Color Enable  **" {
                n180 = Index Array(array=w302, index=4) -> (element=w303:cluster{string[]})
                n181 = call <vilib>:"NT Read String.vi"("Name"=w305) -> ("String"=w304:string)  [unwired: 9 in, 1 out]
                n182 = Unbundle(w303) -> (w299:string[])
                n183 = Match First String(2:w299, 3:w304) -> (0:w300:i32)  [unwired: 1 out]
                n184 = property on="Test Ring" class="Ring (strict)"("Value"=w300, "Strings []"=w299) -> ()  [unwired: 2 in, 2 out]
                n185 = property on="Test Ring" class="Ring (strict)"("Visible"=TRUE) -> ()  [unwired: 2 in, 2 out]
                n186 = property on="Test Slider" class="Slide (strict)"("Visible"=FALSE) -> ()  [unwired: 2 in, 2 out]
              }
              frame Default {
                n187 = property on="Test Ring" class="Ring (strict)"("Visible"=FALSE) -> ()  [unwired: 2 in, 2 out]
                n188 = property on="Test Slider" class="Slide (strict)"("Visible"=FALSE) -> ()  [unwired: 2 in, 2 out]
              }
              frame "Brightness  **", "Color Level  **", "Compression  **", "FPS  **", "Sharpness  **" {
                n189 = call <vilib>:"NT Read Number.vi"("Name"=w311) -> ("Numeric"=w310:dbl)  [unwired: 9 in, 1 out]
                n190 = local write "Test Slider"(w310) -> ()
                n191 = property on="Test Slider" class="Slide (strict)"("Visible"=TRUE, "Scale.Maximum"=100.0 ("Scale.Range:Maximum")) -> ()  [unwired: 2 in, 2 out]
                n192 = property on="Test Ring" class="Ring (strict)"("Visible"=FALSE) -> ()  [unwired: 2 in, 2 out]
              }
            }
          }
        }
        n193 = property on="Progress" class="Clust (strict)"("Visible"=FALSE) -> ()  [unwired: 2 in, 2 out]
      }
      event "Test Name": Mouse Enter {
        # "Populate the ring with the list of tests"
        n194 = event-data() -> ()  [unwired: 1 in, 1 out]
        n195 = call <vilib>:"NT Read String Array.vi"("Name"="/TestMode/TestList") -> ("String Array"=w320:string[])  [unwired: 9 in, 1 out]
        n196 = Build Array (concatenate)("Select the test to run...", w320) -> (w319:string[])
        n197 = property on="Test Name" class="Ring (strict)"("Strings []"=w319) -> ()  [unwired: 2 in, 2 out]
      }
      event "Test Name": Value Change {
        w323 = FALSE ("Visible")
        # "Tell the robot the test name to run"
        n198 = event-data() -> ("NewVal"=w327:u16)  [unwired: 1 in]
        n199 = property on="Test Name" class="Ring (strict)"() -> ("Strings []"=w328:string[])  [unwired: 2 in, 2 out]
        n200 = local write "Progress"(T7 {"Test Progress"=0, "Test Progress Text"=""} ("Progress")) -> ()
        n201 = Index Array(array=w328, index=w327) -> (element=w326:string)
        n202 = call <vilib>:"NT Write String.vi"("String"=w326, "Name"="/TestMode/TestName") -> ()  [unwired: 9 in, 1 out]
        n203 = property on="Progress" class="Clust (strict)"("Visible"=TRUE) -> ()  [unwired: 2 in, 2 out]
        n204 = property on="Motor" class="Clust (strict)"("Visible"=w323) -> ()  [unwired: 2 in, 2 out]
        n205 = property on="Test Slider" class="Slide (strict)"("Visible"=w323) -> ()  [unwired: 2 in, 2 out]
        n206 = property on="On/Off" class="Bool (strict)"("Visible"=w323) -> ()  [unwired: 2 in, 2 out]
        n207 = property on="Rev/Fwd" class="Clust (strict)"("Visible"=w323) -> ()  [unwired: 2 in, 2 out]
        n208 = property on="Test Ring" class="Ring (strict)"("Visible"=w323) -> ()  [unwired: 2 in, 2 out]
      }
      event "Select Auto": Mouse Enter {
        # "Populate the combo box with the list of autonomous options"
        n209 = event-data() -> ()  [unwired: 1 in, 1 out]
        n210 = call <vilib>:"NT Read String Array.vi"("Name"="Auto List") -> ("String Array"=w330:string[])  [unwired: 9 in, 1 out]
        n211 = property on="Select Auto" class="CmbBox"("Strings[]"=w330) -> ()  [unwired: 2 in, 2 out]
      }
      event "Select Auto": Value Change {
        # "User modified the Auto Selection. Write to NT variable so robot knows."
        n212 = event-data() -> ("NewVal"=w334:string)  [unwired: 1 in]
        n213 = call <vilib>:"NT Write String.vi"("String"=w334, "Name"="Auto Selector") -> ()  [unwired: 9 in, 1 out]
      }
      event "Command Selection": Value Change {
        # "Get the params and show in table"
        n214 = event-data() -> ("NewVal"=w341:i32)  [unwired: 1 in]
        n215 = property on="Command Selection" class="MCListbox (strict)"() -> ("ItemNames"=w339:string[][])  [unwired: 2 in, 2 out]
        n216 = call <vilib>:"WPI_DashboardUpdate Command Params.vi"("NewVal"=w341, "Commands"=w339, "Param Tbl"=w340) -> ()  [unwired: 8 in, 1 out]
      }
      event "Execute Command": Value Change {
        # "Started one, Unique ID holds\nresponse"
        n217 = event-data() -> ()  [unwired: 1 in, 1 out]
        n218 = property on="Command Selection" class="MCListbox (strict)"() -> ("ItemNames"=w353:string[][])  [unwired: 2 in, 2 out]
        n219 = Index Array(array=w353, index (row)="Command Selection", index (col)=0) -> (element=w351:string)
        n220 = call <vilib>:"Invoke Commands.vi"("Command Params"="Command Params", "Function Name"=w351) -> ("Params"=w347:u8, "Started"=w346:bool)  [unwired: 7 in, 1 out]
        n221 = Array Subset(array="Command Params", length (row)=w347) -> (w348:string[][])  [unwired: 3 in]
        n222 = Select(t="Executing" ("Cmd Status"), s=w346, f="" ("Cmd Status")) -> (s? t:f=→"Cmd Status":string)
      }
      event "Command Selection": Double Click {
        n223 = event-data() -> ("Row"=w363:i32)  [unwired: 1 in]
        n224 = property on="Command Selection" class="MCListbox (strict)"() -> ("ItemNames"=w366:string[][])  [unwired: 2 in, 2 out]
        n225 = local read "Command Params"() -> (w361:string[][])
        n226 = Index Array(array=w366, index (row)=w363, index (col)=0) -> (element=w364:string)
        n227 = call <vilib>:"Invoke Commands.vi"("Command Params"=w361, "Function Name"=w364) -> ("Params"=w360:u8, "Started"=w355:bool)  [unwired: 7 in, 1 out]
        n228 = Array Subset(array=w361, length (row)=w360) -> (w359:string[][])  [unwired: 3 in]
        n229 = Select(t="Executing" ("Cmd Status"), s=w355, f="" ("Cmd Status")) -> (s? t:f=w356:string)
        n230 = local write "Cmd Status"(w356) -> ()
      }
      event "CheckList": Double Click {
        # "Shift clears all"
        # "Update symbols on the listbox"
        n231 = event-data() -> ("PlatMods.Shift"=w369:bool, "Row"=w371:i32)  [unwired: 1 in]
        n232 = case shown="True" w369 {
          tunnel: w371 -> [w375 _]
          tunnel: 1 -> [w374 _]
          frame False {
            n233 = property on="CheckList" class="LstBox (strict)"() -> ("Item Symbols"=w373:i32[])  [unwired: 2 in, 2 out]
            n234 = Replace Array Subset(array=w373, new element=w374, index=w375) -> (w372:i32[])
            n235 = property on="CheckList" class="LstBox (strict)"("Item Symbols"=w372) -> ()  [unwired: 2 in, 2 out]
          }
          frame True {
            w376 = 0 ("Top Row")
            n236 = property on="CheckList" class="LstBox (strict)"() -> ("Number of Rows"=w378:u32)  [unwired: 2 in, 2 out]
            n237 = Initialize Array(0, w378) -> (w377:i32[])
            n238 = property on="CheckList" class="LstBox (strict)"("Top Row"=w376, "Value"=w376, "Item Symbols"=w377) -> ()  [unwired: 2 in, 2 out]
          }
        }
      }
      event "CheckList": Key Down {
        # "Update symbols on the listbox\nLeft and right keys check and uncheck"
        n239 = event-data() -> ("VKey"=w383:T22)  [unwired: 1 in]
        n240 = case shown="\"Left\", \"Right\"" w383 {
          selector: w383 -> [w388 _]
          tunnel: eventvkey."Left" ("VKey") -> [w386 _]
          frame "Left", "Right" {
            n241 = Equal?(x=w386, y=w388) -> (x = y?=w387:bool)
            n242 = Select(t=0, s=w387, f=1) -> (s? t:f=w389:i32)
            n243 = property on="CheckList" class="LstBox (strict)"() -> ("Item Symbols"=w392:i32[])  [unwired: 2 in, 2 out]
            n244 = Replace Array Subset(array=w392, new element=w389, index="CheckList") -> (w391:i32[])
            n245 = property on="CheckList" class="LstBox (strict)"("Item Symbols"=w391) -> ()  [unwired: 2 in, 2 out]
          }
          frame Default {
          }
        }
      }
      event "DB Camera Config": Value Change {
        # "Show or hide the cluster of controls, store in ini file"
        n246 = event-data() -> ("NewVal"=w397:bool)  [unwired: 1 in]
        n247 = case shown="False" w397 {
          tunnel: w396 -> [w406 _]
          tunnel: [w399 w417] -> w395
          tunnel: w394 -> [w398 w417]
          frame False {
            w413 = "Camera"
            w416 = FALSE ("Visible")
            n248 = local read "Camera Settings"() -> (w405:T2)
            n249 = Index Array(array=w406) -> (element=w409:cluster{string[]})  [unwired: 1 in]
            n250 = Unbundle(w405) -> ("Frame Rate"=w404:i32, "Compression"=w403:i32, "Size"=w407:u16)
            n251 = Unbundle(w409) -> (w408:string[])
            n252 = Index Array(array=w408, index=w407) -> (element=w402:string)
            n253 = call-poly <vilib>:"Write Key.vi"("section"=w413, "value"=w402, "key"="Size", "refnum"=w398) -> ("refnum out"=w415:T20)  [unwired: 2 in, 5 out]
            n254 = call-poly <vilib>:"Write Key.vi"("section"=w413, "value"=w404, "key"="FrameRate", "refnum"=w415) -> ("refnum out"=w414:T20)  [unwired: 1 in, 6 out]
            n255 = property on="Camera Settings" class="Clust (strict)"("Visible"=w416) -> ()  [unwired: 2 in, 2 out]
            n256 = local write "DB Camera Config"(w416) -> ()
            n257 = call-poly <vilib>:"Write Key.vi"("section"=w413, "value"=w403, "key"="Compression", "refnum"=w414) -> ("refnum out"=w400:T20)  [unwired: 1 in, 6 out]
            n258 = call <vilib>:"Close Config Data.vi"("refnum"=w400) -> ("file path"=w401:path)  [unwired: 2 in, 8 out]
            n259 = call <vilib>:"Open Config Data.vi"("configuration file path"=w401) -> ("refnum"=w399:T20)  [unwired: 8 in, 2 out]
          }
          frame True {
            n260 = property on="Camera Settings" class="Clust (strict)"("Visible"=TRUE) -> ()  [unwired: 2 in, 2 out]
          }
        }
      }
      event "Camera Settings": Value Change {
        # "Update summary string when any elements of DB camera change"
        n261 = event-data() -> ("NewVal"=w431:T2)  [unwired: 1 in]
        n262 = Index Array(array=w427) -> (element=w426:cluster{string[]})  [unwired: 1 in]
        n263 = Unbundle(w431) -> ("Frame Rate"=w422:i32, "Compression"=w421:i32, "Size"=w424:u16)
        n264 = Unbundle(w426) -> (w425:string[])
        n265 = Index Array(array=w425, index=w424) -> (element=w423:string)
        n266 = Format Into String(format string="%s   %dfps   %d%%", w423, w422, w421) -> (resulting string=w428:string)  [unwired: 2 in, 1 out]
        n267 = Build Array(w428) -> (w429:string[])
        n268 = property on="DB Camera Config" class="Bool (strict)"("Strings [4]"=w429) -> ()  [unwired: 2 in, 2 out]
      }
      event "Motor.Enable": Value Change {
        # "When the test mode otor enable helper is set, update that\ntree row item's value"
        n269 = event-data() -> ("NewVal"=w438:bool)  [unwired: 1 in]
        n270 = Unbundle("Motor") -> ("Value"=w437:dbl)  [unwired: 1 out]
        n271 = Select(t=w437, s=w438, f=0.0) -> (s? t:f=w435:dbl)
        n272 = call <vilib>:"NT Write Number.vi"("Numeric"=w435, "Name"=w434) -> ()  [unwired: 9 in, 1 out]
      }
      event "Test Slider": Value Change {
        # "When the test mode slider helper is set, update that\ntree row item's value"
        n273 = event-data() -> ("NewVal"=w442:dbl)  [unwired: 1 in]
        n274 = call <vilib>:"NT Write Number.vi"("Numeric"=w442, "Name"=w443) -> ()  [unwired: 9 in, 1 out]
      }
      event "On/Off": Value Change {
        # "When the test mode on/off helper value is set, update that\ntree row item's value"
        n275 = event-data() -> ("NewVal"=w448:bool)  [unwired: 1 in]
        n276 = Boolean To (0,1)(Boolean=w448) -> (0, 1=w447:i16)
        n277 = call <vilib>:"NT Write Number.vi"("Numeric"=w447, "Name"=w446) -> ()  [unwired: 9 in, 1 out]
      }
      event "Rev/Fwd": Value Change {
        # "When the test mode helper value for relays is set, update that\ntree row item's value"
        n278 = event-data() -> ("NewVal.Forward"=w457:bool, "NewVal.Reverse"=w456:bool)  [unwired: 1 in]
        n279 = Boolean To (0,1)(Boolean=w457) -> (0, 1=w453:i16)
        n280 = Boolean To (0,1)(Boolean=w456) -> (0, 1=w455:i16)
        n281 = Negate(x=w455) -> (-x=w454:i16)
        n282 = Add(x=w453, y=w454) -> (x+y=w452:i16)
        n283 = call <vilib>:"NT Write Number.vi"("Numeric"=w452, "Name"=w451) -> ()  [unwired: 9 in, 1 out]
      }
      event "Test Ring": Value Change {
        # "When a test mode helper value is selected from the ring,\nset the tree item's variable to the string value"
        n284 = event-data() -> ("NewVal"=w462:u16)  [unwired: 1 in]
        n285 = property on="Test Ring" class="Ring (strict)"() -> ("Strings []"=w463:string[])  [unwired: 2 in, 2 out]
        n286 = Index Array(array=w463, index=w462) -> (element=w461:string)
        n287 = call <vilib>:"NT Write String.vi"("String"=w461, "Name"=w460) -> ()  [unwired: 9 in, 1 out]
      }
      event "Rec Mode": Value Change {
        # "Update globals for recording mode and path to read log from.\nClear when logging and let NetworkTables set path for vision to\nuse."
        n288 = event-data() -> ("NewVal"=w475:enum32{"Stop", "Record", "Playback"})  [unwired: 1 in]
        n289 = global write "WPI_DashboardLogging Global.vi" "Logging Filename"(path "") -> ()
        n290 = global write "WPI_DashboardLogging Global.vi" "Recording"(w475) -> ()
        n291 = case shown="\"Playback\"" w475 {
          tunnel: w474 -> [_ w477 w486]
          tunnel: [_ _ w485] -> w471
          tunnel: [_ _ w484] -> _
          tunnel: w469 -> [_ _ w482]
          tunnel: cluster{i32, i32} {-250, 170} -> [_ _ w481]
          tunnel: [_ _ T23 {"Image Size"=TRUE, "Image Type"=TRUE, "Pixel Value"=TRUE, "ROI Information"=TRUE, "Zoom Factor"=FALSE} ("Image Information Shown:All Elements")] -> w467
          tunnel: [_ _ TRUE ("Zoom Factor")] -> w466
          tunnel: w465 -> [_ _ w478]
          frame Default {
          }
          frame "Stop", "Record" {
            # "Place Window too"
            n292 = invoke class="VI" method="FP.Close"(reference=w477) -> (reference out=w476:refnum<vi>)  [unwired: 2 in, 2 out]
            n293 = invoke class="VI" method="Abort VI"(reference=w476) -> ()  [unwired: 2 in, 3 out]
          }
          frame "Playback" {
            n294 = call "Open Playback Panel.vi"("Offset"=w481, "DB VI Ref"=w482, "Playback in"=w486) -> ("Playback out"=w483:refnum<vi>)  [unwired: 8 in]
            n295 = register-events(w483, w478) -> (reference out=w485:refnum<event-registration>, error out=w484:errorcluster)  [unwired: 2 in]
          }
        }
        n296 = property on="Camera Image" class="ImageControl"("Image Information Shown"=w467, "Image Information Visible"=w466) -> ()  [unwired: 2 in, 2 out]
        n297 = call <vilib>:"WPI_DashboardNT Log FieldName Cache.vi"("Operation"=enum16{"Lookup/Add", "Index", "Clear"}."Clear") -> ()  [unwired: 8 in, 3 out]
      }
      event Panel Close {
        w488 = enum32{"Stop", "Record", "Playback"}."Stop" ("Rec Mode")
        # "Playback window has been closed, abort"
        n298 = event-data() -> ()  [unwired: 1 in, 4 out]
        n299 = local write "Rec Mode"(w488) -> ()
        n300 = global write "WPI_DashboardLogging Global.vi" "Recording"(w488) -> ()
      }
      event Panel Close {
        # "Abort playback window and ourself"
        n301 = event-data() -> ()  [unwired: 1 in, 4 out]
        n302 = invoke class="VI" method="FP.Close"(reference=w494) -> (reference out=w493:refnum<vi>)  [unwired: 2 in, 2 out]
        n303 = invoke class="VI" method="Abort VI"(reference=w493) -> (error out=w492:errorcluster)  [unwired: 2 in, 2 out]
        n304 = invoke class="VI" method="Abort VI"(error in=w492) -> ()  [unwired: 2 in, 3 out]
      }
      event User Event {
        n305 = event-data() -> ("IDs"=w502:cluster{"RPC field ID":u16, "Unique ID":u16}, "String"=w501:string)  [unwired: 1 in]
        n306 = Bundle("IDs"=w502, "String"=w501) -> (w500:T9)  [unwired: 1 in]
        n307 = call <vilib>:"Retrieve RPC Response.vi"("RPC Response"=w500) -> ("Output"=w497:string[][])  [unwired: 10 in]
        n308 = Build Array (concatenate)(w495, w497) -> (w496:string[][])
        n309 = local write "Command Params"(w496) -> ()
        n310 = local write "Cmd Status"("" ("Cmd Status")) -> ()
      }
      event "Vision": Value Change {
        # "Enable/Disable Compression slider.\nHW USB is hard-coded into the camera"
        n311 = event-data() -> ("NewVal"=w509:u16)  [unwired: 1 in]
        n312 = Equal?(x=w509, y=u32 2 ("milliseconds to wait")) -> (x = y?=w507:bool)
        n313 = Select(t=T24."Disabled and Grayed Out" ("Disabled"), s=w507, f=T24."Enabled" ("Disabled")) -> (s? t:f=w504:T24)
        n314 = property on="Compression" class="Slide (strict)"("DisabledEnum"=w504) -> ()  [unwired: 2 in, 2 out]
      }
      event "Tree": Double Click {
        n315 = event-data() -> ("PlatMods"=w514:T27, "Tag"=w513:string)  [unwired: 1 in]
        n316 = Unbundle(w514) -> ("Shift"=w512:bool)  [unwired: 4 out]
        n317 = Not(x=w512) -> (.not. x?=w511:bool)
        n318 = call <vilib>:"NT Update Persistence.vi"("Persistence"=w511, "Name"=w513) -> ()  [unwired: 9 in, 1 out]
      }
    }
  }
  n319 = while {
    tunnel: w49 -> [w518]
    i -> [w521]
    stop <- FALSE stop-if-true
    n320 = Wait (ms)(milliseconds to wait=u32 100) -> ()  [unwired: 1 out]
    n321 = case shown="\"Playback\"" "Rec Mode" {
      tunnel: w521 -> [_ _ w536]
      tunnel: [u32 2829099 ("Base Color") u32 11141120 ("Target Color") w525] -> w517
      frame "Stop", Default {
        # "Reset the color, extra updates don't cost much"
      }
      frame "Record" {
      }
      frame "Playback" {
        # "Playback"
        n322 = Quotient & Remainder(x=w536, y=u32 50 ("milliseconds to wait")) -> (x-y*floor(x/y)=w532:u32)  [unwired: 1 out]
        n323 = Divide(x=w532, y=u32 50 ("milliseconds to wait")) -> (x/y=w529:dbl)
        n324 = Multiply(x=6.283185307179586, y=w529) -> (x*y=w534:dbl)
        n325 = Sine(x=w534) -> (sin(x)=w533:dbl)
        n326 = Absolute Value(x=w533) -> (abs(x)=w526:dbl)
        n327 = call "Interpolate RGB Color.vi"("Proportion"=w526, "Target Color"=u32 30976, "Base Color"=u32 2829099) -> ("Result Color"=w525:u32)  [unwired: 8 in]
      }
    }
    n328 = property class="Pane"(reference=w518, "PaneColor"=w517) -> ()  [unwired: 1 in, 2 out]
  }
  n329 = while {
    shift-right: [w537] -> w2
    shift-left: w1 -> [w543]
    stop <- FALSE ("stop") stop-if-true
    n330 = call <vilib>:"SD Read Number.vi"("Name"="Hcenter") -> ("Numeric"=w538:dbl)  [unwired: 8 in, 2 out]
    n331 = Wait (ms)(milliseconds to wait=u32 500) -> ()  [unwired: 1 out]
    n332 = call "LightControl.vi"("error in (no error)"=w543, "X"=w538) -> ("error out"=w540:errorcluster)  [unwired: 9 in]
    n333 = call <vilib>:"Clear Errors.vi"("error in (no error)"=w540) -> ("error out"=w537:errorcluster)  [unwired: 5 in, 1 out]
  }
  n334 = local write "Dashboard Tab"(T1."Drive" ("Dashboard Tab")) -> ()
  n335 = call "Shutdown.vi"("error in (no error)"=w2) -> ()  [unwired: 10 in, 1 out]
  n336 = property on="On/Off" class="Bool (strict)"("Visible"=w17) -> ()  [unwired: 2 in, 2 out]
  n337 = property on="Motor" class="Clust (strict)"("Visible"=w17) -> ()  [unwired: 2 in, 2 out]
  n338 = property on="Progress" class="Clust (strict)"("Visible"=w17) -> ()  [unwired: 2 in, 2 out]
  n339 = property on="Test Ring" class="Ring (strict)"("Visible"=w17) -> ()  [unwired: 2 in, 2 out]
  n340 = property on="Rev/Fwd" class="Clust (strict)"("Visible"=w17) -> ()  [unwired: 2 in, 2 out]
  n341 = property on="Camera Settings" class="Clust (strict)"("Visible"=w17) -> ()  [unwired: 2 in, 2 out]
  n342 = while {
    tunnel: u16 1741 ("timeout ms (25000)") -> [w545]
    stop <- FALSE stop-if-true
    n343 = TCP Create Listener(10:w545) -> (0:w544:errorcluster, 3:w546:refnum<k5>)  [unwired: 4 in, 1 out]
    n344 = case shown="No Error" w544 {
      selector: w544 -> [w548 _]
      tunnel: w546 -> [w549 _]
      frame No Error {
        n345 = while {
          tunnel: w549 -> [w552]
          tunnel: w548 -> [w551]
          stop <- FALSE stop-if-true
          n346 = TCP Wait On Listener(8:w551, 11:w552) -> (0:w553:errorcluster, 4:w554:refnum<k5>)  [unwired: 2 in, 3 out]
          n347 = local write "TCP"(w554) -> ()
          n348 = case shown="No Error" w553 {
            frame No Error {
            }
            frame Error {
              n349 = Wait (ms)(milliseconds to wait=u32 1000) -> ()  [unwired: 1 out]
            }
          }
        }
      }
      frame Error {
        n350 = Wait (ms)(milliseconds to wait=u32 1000) -> ()  [unwired: 1 out]
      }
    }
  }
  n351 = local write "DB Camera Config"(w17) -> ()
  n352 = local write "Command Params"(string[][] [] ("Command Params")) -> ()
  n353 = global write "WPI_DashboardLogging Global.vi" "Recording"(w43) -> ()
  n354 = local write "Command Selection"(u16 0 ("milliseconds to wait")) -> ()
  n355 = local write "Rec Mode"(w43) -> ()
